vi "parse_PoseStamped.vi"(8 "error in":errorcluster, 11 "msg in":string) -> (0 "error out":errorcluster, 2 "PoseStamped":T1, 3 "msg out":string)   [LabVIEW 2012]
doc: "Parses a message into a stamped pose"
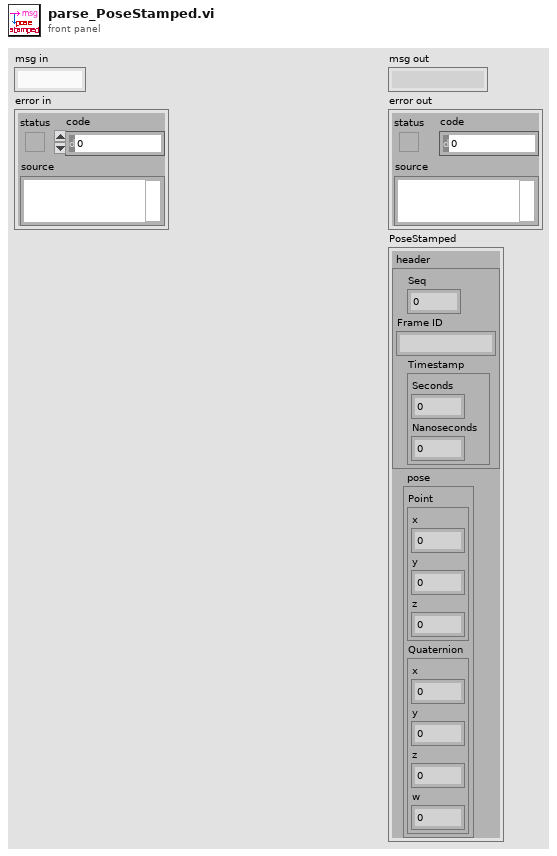
[diagram p1: front panel]
types:
  T1 = cluster{" header":cluster{"Seq":u32, "Frame ID":string, "Timestamp":cluster{"Seconds":i32, "Nanoseconds":i32}}, " pose":cluster{"Point":cluster{"x":dbl, "y":dbl, "z":dbl}, "Quaternion":cluster{"x":dbl, "y":dbl, "z":dbl, "w":dbl}}}
  T2 = cluster{"Seq":u32, "Frame ID":string, "Timestamp":cluster{"Seconds":i32, "Nanoseconds":i32}}
  T3 = cluster{"Point":cluster{"x":dbl, "y":dbl, "z":dbl}, "Quaternion":cluster{"x":dbl, "y":dbl, "z":dbl, "w":dbl}}
  T4 = cluster{"Header":cluster{"Seq":u32, "Frame ID":string, "Timestamp":cluster{"Seconds":i32, "Nanoseconds":i32}}, "Pose":cluster{"Point":cluster{"x":dbl, "y":dbl, "z":dbl}, "Quaternion":cluster{"x":dbl, "y":dbl, "z":dbl, "w":dbl}}}
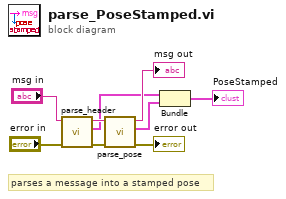
[diagram p0: block diagram]
diagram:
  # "parses a message into a stamped pose"
  n1 = call "parse_header.vi"("error in"="error in", "msg in"="msg in") -> ("error out"=w6:errorcluster, "Header"=w3:T2, "msg out"=w7:string)  [unwired: 3 in]
  n2 = call "parse_pose.vi"("error in"=w6, "msg in"=w7) -> ("error out"=→"error out":errorcluster, "Pose"=w2:T3, "msg out"=→"msg out":string)  [unwired: 3 in]
  n3 = Bundle("Header"=w3, "Pose"=w2) -> (→"PoseStamped":T4)  [unwired: 1 in]
